vi "Throughput Calculation.vi"(11 "Data":u32[](array[numeric])) -> (1 "Average Throughput":cluster{"mean":dbl, "mean":dbl}(graph), 2 "Inst. PXI Throughput":dbl format="%#_6p", 3 "Inst. Disk Write Throughput":dbl format="%#_6p", 5 "Loop Time":u32=50)   [LabVIEW 2012]
uses:
  <vilib>/ptbypt/NI_PtbyPt.lvlib
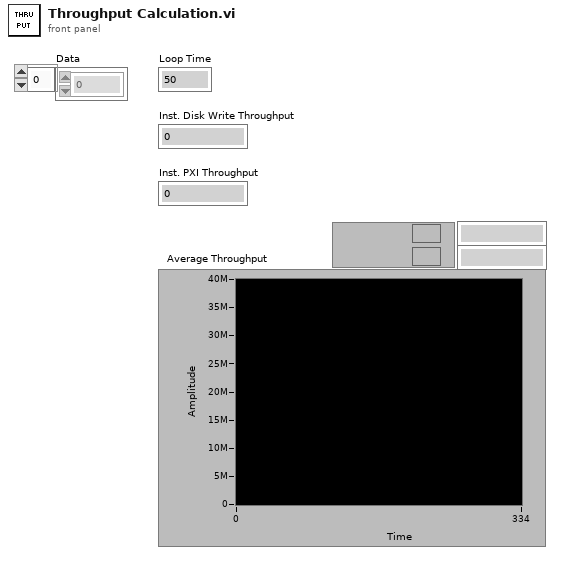
[diagram p1: front panel]
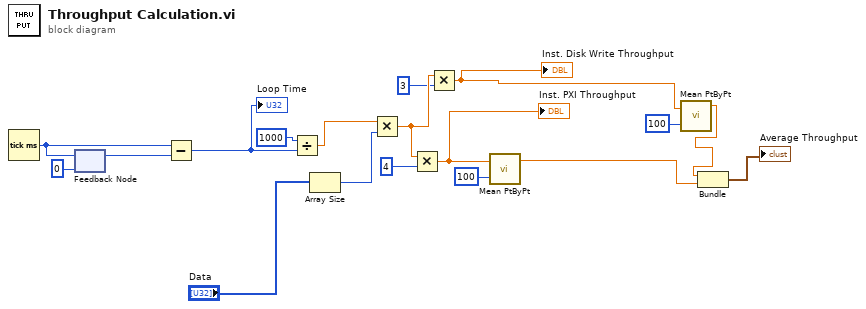
[diagram p0: block diagram]
diagram:
  n1 = Tick Count (ms)() -> (millisecond timer value=w16:u32)
  n2 = feedback #1(u32 0 ("millisecond timer value")) -> (w17:u32)
  n3 = feedback-in #1(w16) -> ()
  n4 = Subtract(x=w16, y=w17) -> (x-y=w3:u32)
  "Loop Time" <- w3
  n5 = Divide(x=u32 1000, y=w3) -> (x/y=w8:dbl)
  n6 = Array Size(array="Data") -> (size(s)=w7:i32)
  n7 = Multiply(x=w8, y=w7) -> (x*y=w10:dbl)
  n8 = Multiply(x=w10, y=4) -> (x*y=w5:dbl)
  "Inst. PXI Throughput" <- w5
  n9 = Multiply(x=w10, y=3) -> (x*y=w12:dbl)
  "Inst. Disk Write Throughput" <- w12
  n10 = call <vilib>:"Mean PtByPt.vi"("x"=w5, "sample length"=100) -> ("mean"=w14:dbl)  [unwired: 2 in, 1 out]
  n11 = call <vilib>:"Mean PtByPt.vi"("x"=w12, "sample length"=100) -> ("mean"=w13:dbl)  [unwired: 2 in, 1 out]
  n12 = Bundle("mean"=w13, "mean"=w14) -> (→"Average Throughput":cluster{"mean":dbl, "mean":dbl})  [unwired: 1 in]
